vi "JTAG Config.vi"(8 "error in (no error)":errorcluster, 11 "Function":u16(ring)=5 items=["Initialize COMMs", "Release COMMs", "Initialize Variables", "Select 1MHz DCO", "Select 8MHz DCO", "Standard Startup"]) -> (0 "error out":errorcluster)   [LabVIEW 2009]
panel:
  out "PC start address":u16=14304 format="%04x"
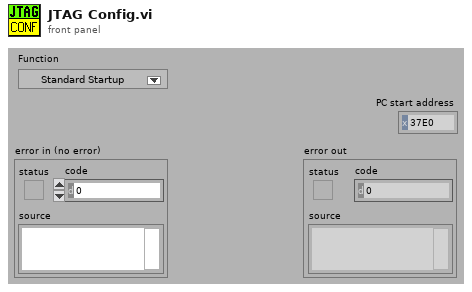
[diagram p1: front panel]
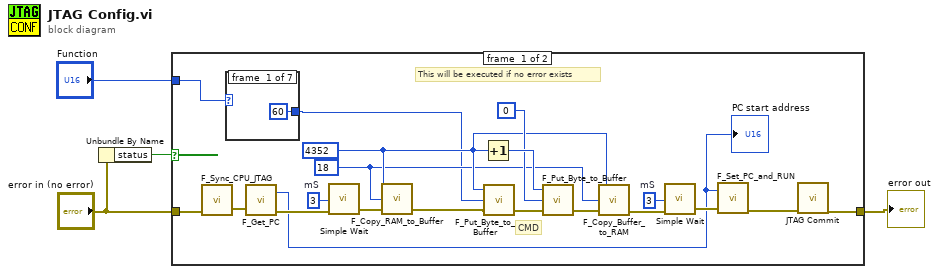
[diagram p0: block diagram]
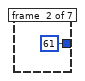
[diagram p2: hidden frame]
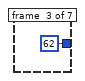
[diagram p3: hidden frame]
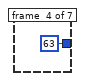
[diagram p4: hidden frame]
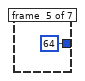
[diagram p5: hidden frame]
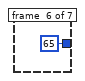
[diagram p6: hidden frame]
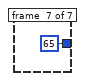
[diagram p7: hidden frame]
diagram:
  n1 = Unbundle By Name("error in (no error)") -> ("status"=w3:bool)
  n2 = case shown="False" w3 {
    tunnel: [w8 w32] -> w4
    tunnel: "error in (no error)" -> [w9 w32]
    tunnel: "Function" -> [w12 _]
    frame #0 {
      w19 = u32 3  # mS
      w20 = u32 3  # mS
      w15 = u16 18
      w16 = u16 4352
      # "CMD"
      # "This will be executed if no error exists"
      n3 = call "F_Sync_CPU_JTAG.vi"("error in (no error)"=w9) -> ("error out"=w7:errorcluster)  [unwired: 1 in, 1 out]
      n4 = case shown="6" w12 {
        tunnel: [60 61 62 63 64 65 65] -> w10
        frame #0 {
        }
        frame #1 {
        }
        frame #2 {
        }
        frame #3 {
        }
        frame #4 {
        }
        frame #5 {
        }
        frame #6 {
        }
      }
      n5 = call "F_Get_PC.vi"("error in (no error)"=w7) -> ("error out"=w6:errorcluster, "Program Counter"=w5:u16)  [unwired: 1 in]
      "PC start address" <- w5
      n6 = call "Simple Wait.vi"("mS"=w20, "error in"=w6) -> ("error out"=w17:errorcluster)  [unwired: 12 in, 1 out]
      n7 = call "F_Copy_RAM_to_Buffer.vi"("error in (no error)"=w17, "Block size to be copied"=w15, "RAM start address"=w16) -> ("error out"=w14:errorcluster)  [unwired: 2 in]
      n8 = Increment(x=w16) -> (x+1=w23:u16)
      n9 = call "F_Put_Byte_to_Buffer.vi"("error in (no error)"=w14, "New value"=w10, "Address of byte to be updated"=w16) -> ("error out"=w24:errorcluster)  [unwired: 2 in]
      n10 = call "F_Put_Byte_to_Buffer.vi"("error in (no error)"=w24, "New value"=u16 0, "Address of byte to be updated"=w23) -> ("error out"=w21:errorcluster)  [unwired: 2 in]
      n11 = call "F_Copy_Buffer_to_RAM.vi"("error in (no error)"=w21, "Block size to be copied"=w15, "Buffer start address"=w16) -> ("error out"=w18:errorcluster)  [unwired: 2 in]
      n12 = call "Simple Wait.vi"("mS"=w19, "error in"=w18) -> ("error out"=w13:errorcluster)  [unwired: 12 in, 1 out]
      n13 = call "F_Set_PC_and_RUN.vi"("error in (no error)"=w13, "PC start address"=w5) -> ("error out"=w11:errorcluster)  [unwired: 1 in]
      n14 = call "JTAG Commit.vi"("error in (no error)"=w11) -> ("error out"=w8:errorcluster)  [unwired: 10 in]
    }
    frame #1 {
      # "Error exists, skip all functions"
    }
  }
  "error out" <- w4
